vi "FTW-Producer-Enqueue.vi"(0 "FTW-Producer In":refnum<class "FTW-Producer.lvclass">, 5 "Header":string, 7 "Body":string, 9 "Timeout":i32=1000 format="%dmsec", 11 "error in":errorcluster) -> (4 "FTW-Producer Out":refnum<class "FTW-Producer.lvclass">, 10 "Timed out?":bool, 14 "Send Time":dbl format="%.6fsec", 15 "error out":errorcluster)   [LabVIEW 2013, in "FTW-Producer.lvclass"]
uses:
  FTW-Producer.lvclass
  FTW-Producer.lvclass/FTW-Producer.ctl
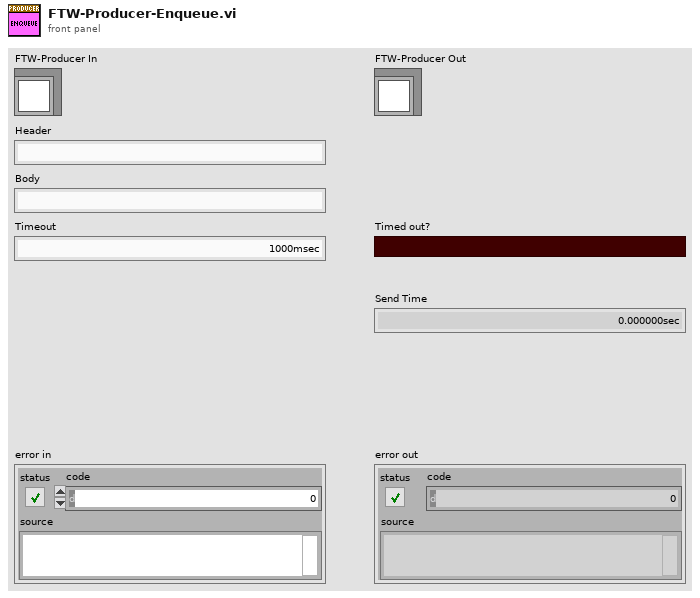
[diagram p1: front panel]
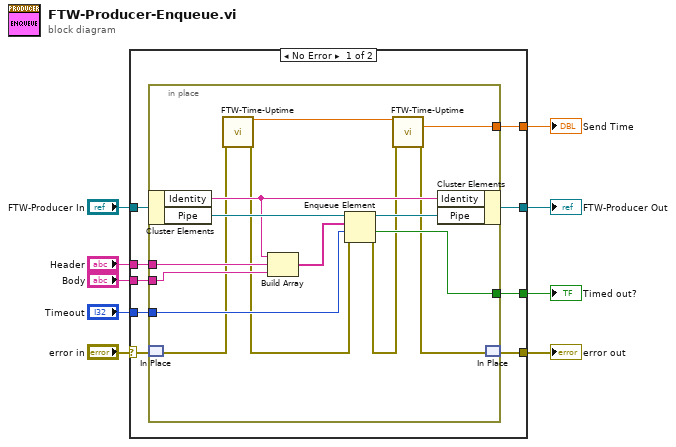
[diagram p0: block diagram]
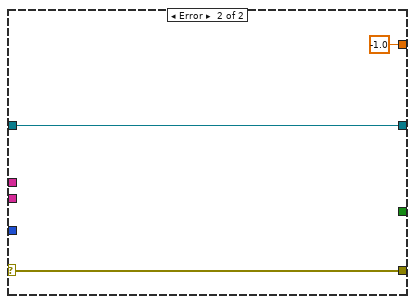
[diagram p2: hidden frame]
diagram:
  n1 = case shown="No Error" "error in" {
    selector: "error in" -> [w16 w35]
    tunnel: [w15 w35] -> w6
    tunnel: [w17 w34] -> w8
    tunnel: "FTW-Producer In" -> [w18 w34]
    tunnel: "Header" -> [w14 _]
    tunnel: "Body" -> [w13 _]
    tunnel: "Timeout" -> [w12 _]
    tunnel: [w11 _] -> w2
    tunnel: [w10 -1.0 ("Elapsed Time")] -> w1
    frame No Error {
      n2 = in-place {
        in-place-border: w14 -> [w30]
        in-place-border: w13 -> [w29]
        in-place-border: w12 -> [w26]
        in-place-border: [w25] -> w11
        in-place-border: [w24] -> w10
        n3 = in-place-cluster #1(w18) -> ("Identity"=w28:string, "Pipe"=w32:refnum<queue>)
        n4 = in-place-match #2(w16) -> (w23:errorcluster)
        n5 = call "FTW-Time-Uptime.vi"("error in"=w23) -> ("Current Uptime"=w19:dbl, "error out"=w22:errorcluster)  [unwired: 12 in, 1 out]
        n6 = Build Array(w28, w30, w29) -> (w27:string[])
        n7 = Enqueue Element(queue=w32, element=w27, timeout in ms (-1)=w26, error in (no error)=w22) -> (queue out=w31:refnum<queue>, timed out?=w25:bool, error out=w21:errorcluster)
        n8 = call "FTW-Time-Uptime.vi"("Previous Uptime"=w19, "error in"=w21) -> ("Elapsed Time"=w24:dbl, "error out"=w20:errorcluster)  [unwired: 11 in, 1 out]
        n9 = in-place-cluster #1("Identity"=w28, "Pipe"=w31) -> (w17:refnum<class "FTW-Producer.lvclass">)
        n10 = in-place-match #2(w20) -> (w15:errorcluster)
      }
    }
    frame Error {
    }
  }
  "FTW-Producer Out" <- w8
  "error out" <- w6
  "Timed out?" <- w2
  "Send Time" <- w1
